vi "U2000_USB_PM_Configure_Trigger.vi"(0 "VISA resource name":refnum<visa-resource-name>, 1 "Trigger Count (1)":i32=1, 2 "Enable Setting-time Delay (F: Disable)":bool, 5 "Trigger Level (0 dBm)":dbl, 7 "Trigger Slope (0: Positive)":u16(ring) items=["Positive", "Negative"], 9 "Trigger Source (3: Immediate)":i32(ring)=3 items=["Bus", "External", "Hold", "Immediate", "Internal A"], 11 "error in (no error)":errorcluster, 12 "Trigger Hysteresis (0 dB)":dbl) -> (4 "VISA resource name out":refnum<visa-resource-name>, 15 "error out":errorcluster)   [LabVIEW 2015]
doc: "Controls the behavior of the trigger system, including Trigger Source, Trigger Slope,Trigger Level, Trigger Delay, Trigger Count and Hysteresis."
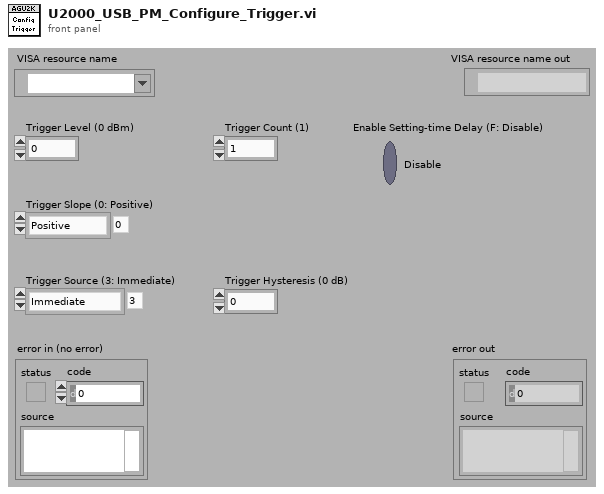
[diagram p1: front panel]
types:
  T1 = typedef "U20xx_USB_PM_User_Data_Out.ctl" = cluster{"U2000 Series Mode":u16, "Trigger Source Int/Ext":bool}
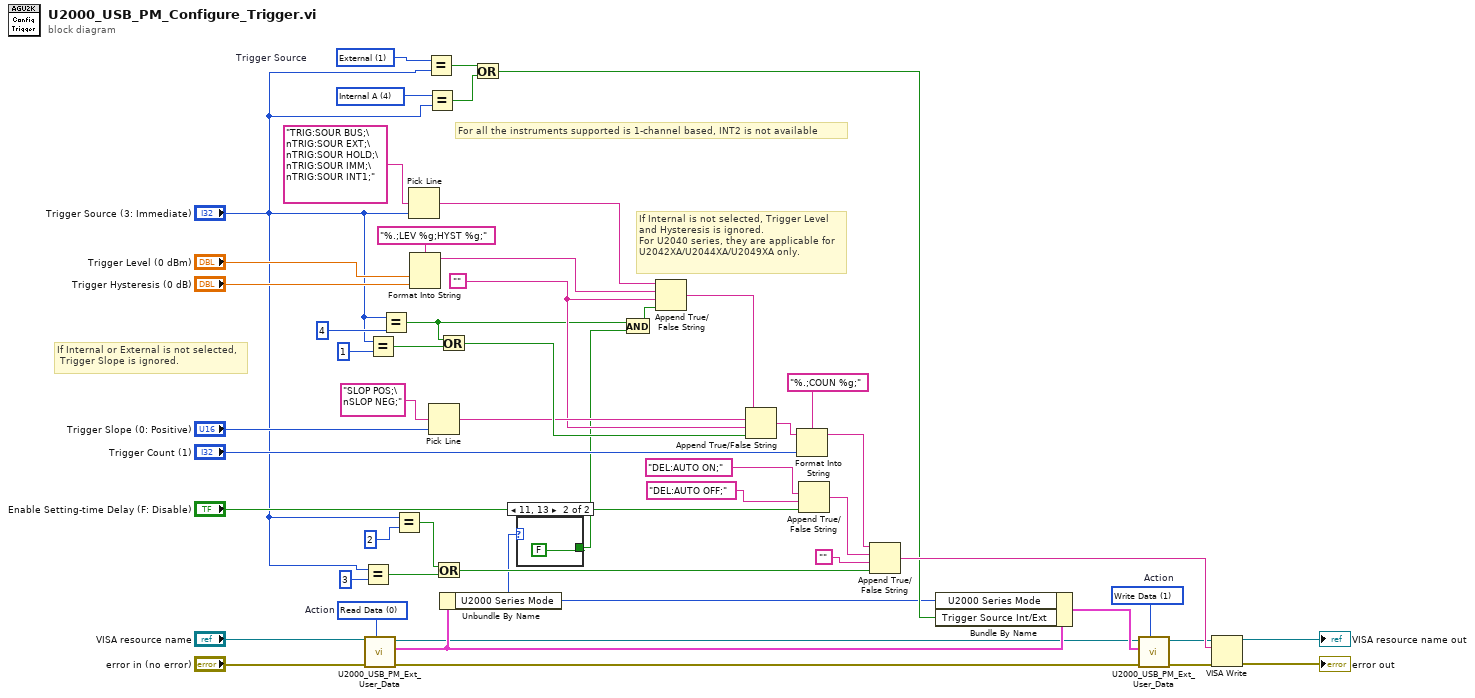
[diagram p0: block diagram]
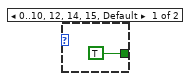
[diagram p2: hidden frame]
diagram:
  w16 = 0 items=["Read Data", "Write Data", "Clear Data", "Clear ALL Data"]  # Action
  w17 = 1 items=["Read Data", "Write Data", "Clear Data", "Clear ALL Data"]  # Action
  w18 = 4 items=["Bus", "External", "Hold", "Immediate", "Internal A"] ("Trigger Source (3: Immediate)")
  w19 = 1 items=["Bus", "External", "Hold", "Immediate", "Internal A"]  # Trigger Source
  w36 = ""
  # "If Internal or External is not selected,\n Trigger Slope is ignored."
  # "If Internal is not selected, Trigger Level and Hysteresis is ignored.\nFor U2040 series, they are applicable for U2042XA/U2044XA/U2049XA only."
  # "For all the instruments supported is 1-channel based, INT2 is not available"
  n1 = Equal?(x="Trigger Source (3: Immediate)", y=3) -> (x = y?=w32:bool)
  n2 = call "U2000_USB_PM_Ext_User_Data.vi"("Action (1: Write Data)"=w16, "error in (no error)"="error in (no error)", "VISA resource name"="VISA resource name") -> ("error out"=w9:errorcluster, "User Data Out"=w12:T1, "VISA resource name out"=w10:refnum<visa-resource-name>)  [unwired: 6 in]
  n3 = Equal?(x="Trigger Source (3: Immediate)", y=1) -> (x = y?=w5:bool)
  n4 = Equal?(x="Trigger Source (3: Immediate)", y=4) -> (x = y?=w4:bool)
  n5 = Equal?(x="Trigger Source (3: Immediate)", y=2) -> (x = y?=w33:bool)
  n6 = Pick Line(multi-line string="TRIG:SOUR BUS;\nTRIG:SOUR EXT;\nTRIG:SOUR HOLD;\nTRIG:SOUR IMM;\nTRIG:SOUR INT1;", line index="Trigger Source (3: Immediate)") -> (output string=w28:string)  [unwired: 1 out]
  n7 = Format Into String(format string="%.;LEV %g;HYST %g;", "Trigger Level (0 dBm)", "Trigger Hysteresis (0 dB)") -> (resulting string=w40:string)  [unwired: 2 in, 1 out]
  n8 = Equal?(x=w19, y="Trigger Source (3: Immediate)") -> (x = y?=w21:bool)
  n9 = Equal?(x=w18, y="Trigger Source (3: Immediate)") -> (x = y?=w20:bool)
  n10 = Pick Line(multi-line string="SLOP POS;\nSLOP NEG;", line index="Trigger Slope (0: Positive)") -> (output string=w38:string)  [unwired: 1 out]
  n11 = Or(x=w33, y=w32) -> (x .or. y?=w31:bool)
  n12 = Or(x=w4, y=w5) -> (x .or. y?=w41:bool)
  n13 = Unbundle By Name(w12) -> ("U2000 Series Mode"=w1:u16)
  n14 = Or(x=w21, y=w20) -> (x .or. y?=w15:bool)
  n15 = case shown="11, 13" w1 {
    tunnel: [TRUE FALSE] -> w2
    frame 0..10, 12, 14, 15, Default {
    }
    frame 11, 13 {
    }
  }
  n16 = And(x=w4, y=w2) -> (x .and. y?=w3:bool)
  n17 = Append True/False String(1:w3, 2:w36, 3:w40, 4:w28) -> (0:w39:string)
  n18 = Append True/False String(1:w41, 2:w36, 3:w38, 4:w39) -> (0:w25:string)
  n19 = Format Into String(format string="%.;COUN %g;", initial string=w25, "Trigger Count (1)") -> (resulting string=w24:string)  [unwired: 1 in, 1 out]
  n20 = Append True/False String(1:"Enable Setting-time Delay (F: Disable)", 2:"DEL:AUTO OFF;", 3:"DEL:AUTO ON;") -> (0:w26:string)  [unwired: 1 out]
  n21 = Append True/False String(1:w31, 2:"", 3:w26, 4:w24) -> (0:w27:string)
  n22 = Bundle By Name(cluster=w12, "U2000 Series Mode"=w1, "Trigger Source Int/Ext"=w15) -> (w11:T1)
  n23 = call "U2000_USB_PM_Ext_User_Data.vi"("Action (1: Write Data)"=w17, "error in (no error)"=w9, "User Data In"=w11, "VISA resource name"=w10) -> ("error out"=w7:errorcluster, "VISA resource name out"=w8:refnum<visa-resource-name>)  [unwired: 5 in, 1 out]
  n24 = VISA Write(VISA resource name=w8, write buffer=w27, error in (no error)=w7) -> (VISA resource name out=→"VISA resource name out":refnum<visa-resource-name>, error out=→"error out":errorcluster)  [unwired: 1 out]
